vi "StellarNet Init, Read, Close.vi"(0 "Integration Time (ms)":i32=100 caption="Inter scan delay ms", 1 "Use Config\nFile Params (T)":bool, 5 "Number of Scans to Average":i32=1 min=1 max=10000 step=1, 7 "Digitizer Clock Rate Setting":i32=3 min=1 max=3, 9 "Optical Smoothing Level":i32=1 min=0 max=4 step=1, 11 "error in (no error)":errorcluster, 12 "Spectral Channel":i32=1 min=0 max=1 step=1, 14 "Temp  Compensation":bool) -> (4 "Spectrum":cluster{"Wavelengths":dbl[], "buffer out":sgl[]}(graph), 6 "output param":i32, 10 "Critical Error":bool, 15 "error out":errorcluster)   [LabVIEW 2023]
panel:
  in  "DLL relative path":path=path "DLL/Swdll.dll"
  in  "Name of SpectraWiz initialization file":path=path "sw.ini"
  in  "Spectrometer Coefficients file":path=path "StellarNet init-read-close coeffs.xml"
  in  "Operating Parameters file":path=path "StellarNet init-read-close parameters.xml"
  out "DLL Path":path
  out "Project Path":path
  # "Use Panel\nParams"
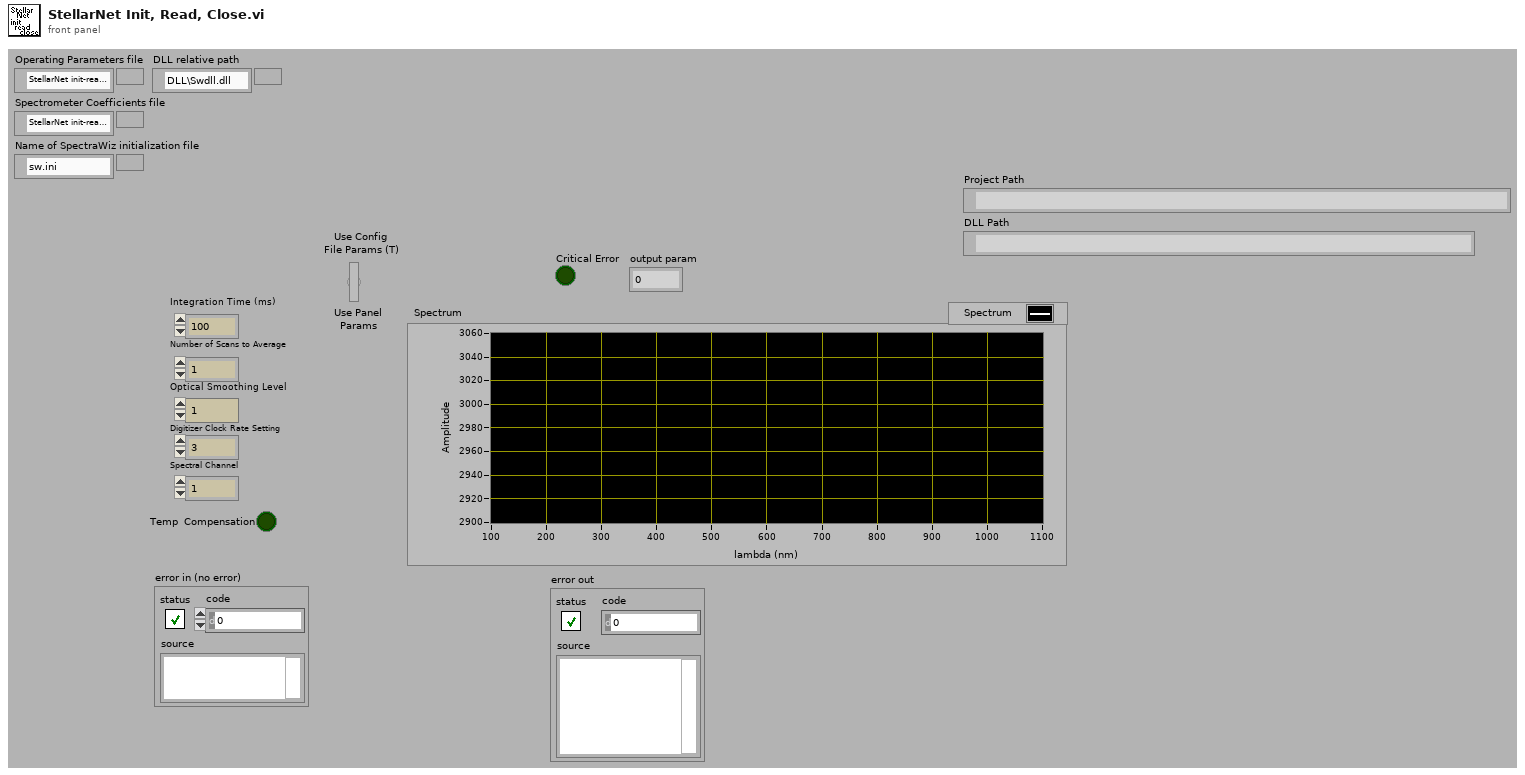
[diagram p1: front panel]
types:
  T1 = cluster{"Coefficients":ext[], "Wavelengths":dbl[]}[]
  T2 = cluster{"Integration Time (ms)":i32, "Number of Scans to Average":i32, "Optical Smoothing Level":i32, "Digitizer Clock Rate Setting":i32, "Temp  Compensation ":bool}[]
  T3 = cluster{"Coefficients":ext[], "Wavelengths":dbl[]}
  T4 = cluster{"Integration Time (ms)":i32, "Number of Scans to Average":i32, "Optical Smoothing Level":i32, "Digitizer Clock Rate Setting":i32, "Temp  Compensation ":bool}
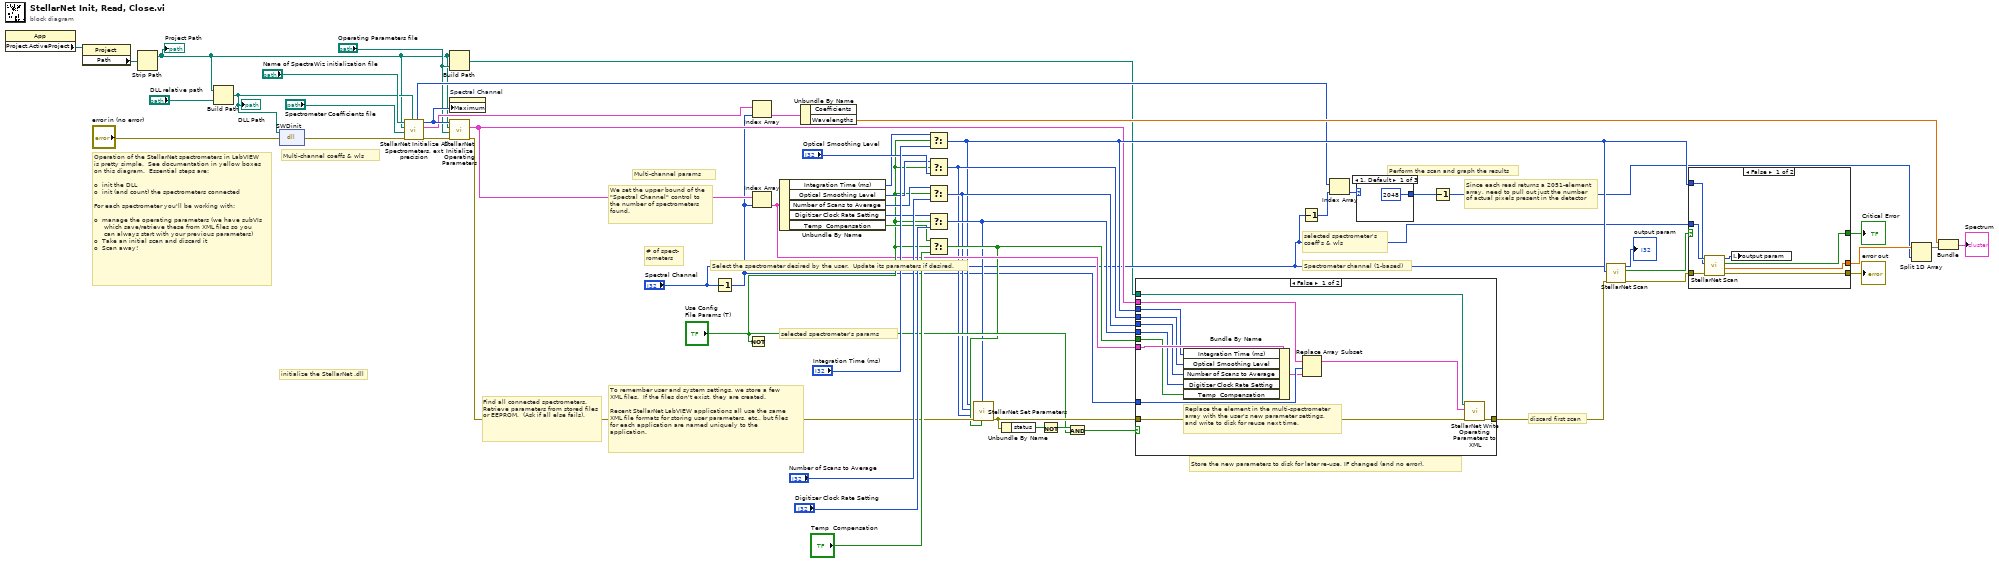
[diagram p0: block diagram]
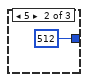
[diagram p2: hidden frame]
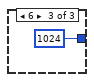
[diagram p3: hidden frame]
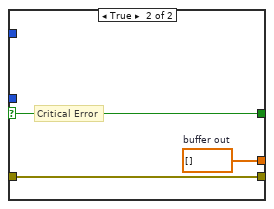
[diagram p5: hidden frame]
diagram:
  # "Operation of the StellarNet spectrometers in LabVIEW\nis pretty simple.  See documentation in yellow boxes\non this diagram.  Essential steps are:\n\no  init the DLL\no  init (and count) the spectrometers connected\n\nFor each spectrometer you'll be working with:\n\no  manage the operating parameters (we have subVIs\n     which save/retrieve these from XML files so you\n     can always start with your previous parameters)\no  Take an initial scan and discard it\no  Scan away!"
  # "initialize the StellarNet .dll"
  # "Since each read returns a 2051-element\narray, need to pull out just the number\nof actual pixels present in the detector"
  # "Spectrometer channel (1-based)"
  # "Perform the scan and graph the results"
  # "We set the upper bound of the\n\"Spectral Channel\" control to \nthe number of spectrometers \nfound."
  # "To remember user and system settings, we store a few \nXML files.  If the files don't exist, they are created.\n\nRecent StellarNet LabVIEW applications all use the same\nXML file formats for storing user parameters, etc., but files\nfor each application are named uniquely to the \napplication."
  # "Store the new parameters to disk for later re-use, IF changed (and no error)."
  # "Select the spectrometer desired by the user.  Update its parameters if desired."
  # "Find all connected spectrometers.  Retrieve parameters from stored files or EEPROM.  (Ask if all else fails)."
  # "selected spectrometer's\ncoeff's & wls"
  # "Multi-channel coeffs & wls"
  # "selected spectrometer's params"
  # "# of spect-\nrometers"
  # "Multi-channel params"
  # "discard first scan"
  n1 = property class="App"() -> ("Project.ActiveProject"=w5:refnum<vi>)  [unwired: 2 in, 2 out]
  n2 = property class="Project"(reference=w5) -> ("Path"=w4:path)  [unwired: 1 in, 2 out]
  n3 = Strip Path(path=w4) -> (stripped path=w1:path)  [unwired: 1 out]
  "Project Path" <- w1
  n4 = Build Path(base path=w1, name or relative path="DLL relative path") -> (appended path=w2:path)
  "DLL Path" <- w2
  n5 = dll-call lib="C:/Program Files/StellarNet/SpectraWiz/swdll.dll" fn="SWDinit" label="init"(path in=w2, error in="error in (no error)") -> (error out=w9:errorcluster)  [unwired: 2 in, 1 out]
  n6 = call "StellarNet Initialize All Spectrometers, ext precision.vi"("Path of swdll.dll"=w2, "error in"=w9, "Spectrometer Coefficients file"="Spectrometer Coefficients file", "Location of SpectraWiz"=w1, "Name of SpectraWiz initialization file"="Name of SpectraWiz initialization file") -> ("error out"=w42:errorcluster, "Multi Channel Coeffs & WLs"=w40:T1, "Number of Channels"=w41:i32, "Detector Types"=w13:u16[])  [unwired: 2 in, 1 out]
  n7 = Build Path(base path=w1, name or relative path="Operating Parameters file") -> (appended path=w7:path)
  n8 = property on="Spectral Channel" class="DigNum (strict)"("Maximum"=w41) -> ()  [unwired: 2 in, 2 out]
  n9 = call "StellarNet Initialize Operating Parameters.vi"("error in"=w42, "Spectrometer Coefficients file"="Operating Parameters file", "Location of SpectraWiz"=w1, "Number of Channels"=w41) -> ("error out"=w38:errorcluster, "Operating Parameters"=w19:T2)  [unwired: 6 in]
  n10 = Decrement(x="Spectral Channel") -> (x-1=w18:i32)
  n11 = Not(x="Use Config\nFile Params (T)") -> ()  [unwired: 1 out]
  n12 = Index Array(array=w40, index=w18) -> (element=w39:T3)
  n13 = Index Array(array=w19, index=w18) -> (element=w25:T4)
  n14 = Unbundle By Name(w25) -> ("Integration Time (ms)"=w36:i32, "Optical Smoothing Level"=w35:i32, "Number of Scans to Average"=w34:i32, "Digitizer Clock Rate Setting"=w33:i32, "Temp  Compensation"=w32:bool)
  n15 = Unbundle By Name(w39) -> ("Wavelengths"=w37:dbl[])  [unwired: 1 out]
  n16 = Select(t=w36, s="Use Config\nFile Params (T)", f="Integration Time (ms)") -> (s? t:f=w20:i32)
  n17 = Select(t=w35, s="Use Config\nFile Params (T)", f="Optical Smoothing Level") -> (s? t:f=w21:i32)
  n18 = Select(t=w34, s="Use Config\nFile Params (T)", f="Number of Scans to Average") -> (s? t:f=w22:i32)
  n19 = Select(t=w33, s="Use Config\nFile Params (T)", f="Digitizer Clock Rate Setting") -> (s? t:f=w23:i32)
  n20 = Select(t=w32, s="Use Config\nFile Params (T)", f="Temp  Compensation") -> (s? t:f=w24:bool)
  n21 = call "StellarNet Set Parameters.vi"("Temp  Compensation"=w24, "Digitizer Clock Rate Setting"=w23, "error in (no error)"=w38, "Optical Smoothing Level"=w21, "Number of Scans to Average"=w22, "Integration Time (ms)"=w20) -> ("error out"=w31:errorcluster)  [unwired: 5 in]
  n22 = Unbundle By Name(w31) -> ("status"=w29:bool)
  n23 = Not(x=w29) -> (.not. x?=w28:bool)
  n24 = And(x=w28, y="Use Config\nFile Params (T)") -> (x .and. y?=w26:bool)
  n25 = case shown="False" w26 {
    tunnel: w31 -> [w57 w69]
    tunnel: [w56 w69] -> w30
    tunnel: w25 -> [w68 _]
    tunnel: w24 -> [w67 _]
    tunnel: w23 -> [w66 _]
    tunnel: w22 -> [w65 _]
    tunnel: w21 -> [w64 _]
    tunnel: w20 -> [w63 _]
    tunnel: w19 -> [w62 _]
    tunnel: w18 -> [w61 _]
    tunnel: w7 -> [w58 _]
    frame False {
      # "Replace the element in the multi-spectrometer\narray with the user's new parameter settings,\nand write to disk for reuse next time."
      n26 = Bundle By Name(cluster=w68, "Integration Time (ms)"=w63, "Optical Smoothing Level"=w64, "Number of Scans to Average"=w65, "Digitizer Clock Rate Setting"=w66, "Temp  Compensation"=w67) -> (w60:T4)
      n27 = Replace Array Subset(array=w62, new element=w60, index=w61) -> (w59:T2)
      n28 = call "StellarNet Write Operating Parameters to XML.vi"("error in (no error)"=w57, "Operating Parameters"=w59, "XML File Path"=w58) -> ("error out"=w56:errorcluster)  [unwired: 8 in]
    }
    frame True {
    }
  }
  n29 = Decrement(x="Spectral Channel") -> (x-1=w15:i32)
  n30 = Index Array(array=w13, index=w15) -> (element=w14:u16)
  n31 = case shown="1, Default" w14 {
    tunnel: [2048 512 1024] -> w11
    frame 1, Default {
    }
    frame 5 {
    }
    frame 6 {
    }
  }
  n32 = Decrement(x=w11) -> (x-1=w10:i32)
  n33 = call "StellarNet Scan.vi"("error in (no error)"=w30, "Integration Time (msec)"=w20, "Spectral Channel"="Spectral Channel") -> ("error out"=w49:errorcluster, "Critical Error"=w50:bool, "output param"=→"output param":i32)  [unwired: 5 in, 1 out]
  n34 = case shown="False" w50 {
    selector: w50 -> [_ w82]
    tunnel: "Spectral Channel" -> [w79 _]
    tunnel: [w78 w81] -> w17
    tunnel: [w76 w82] -> w46
    tunnel: w49 -> [w75 w80]
    tunnel: [w74 w80] -> w48
    tunnel: w20 -> [w73 _]
    frame False {
      n35 = call "StellarNet Scan.vi"("error in (no error)"=w75, "Integration Time (msec)"=w73, "Spectral Channel"=w79) -> ("error out"=w74:errorcluster, "buffer out"=w78:sgl[], "Critical Error"=w76:bool, "output param"=w77:i32)  [unwired: 5 in]
      n36 = local write "output param"(w77) -> ()
    }
    frame True {
      w81 = sgl[] []  # buffer out
      # "Critical Error"
    }
  }
  "error out" <- w48
  "Critical Error" <- w46
  n37 = Split 1D Array(array=w17, index=w10) -> (first subarray=w16:sgl[])  [unwired: 1 out]
  n38 = Bundle("Wavelengths"=w37, w16) -> (→"Spectrum":cluster{"Wavelengths":dbl[], sgl[]})  [unwired: 1 in]
